vi "CLSUIP_ClearBlockDiagram.vi"(8 "error in (no error)":errorcluster, 11 "VI Refnum":refnum<vi>) -> (0 "error out":errorcluster, 3 "VI Refnum out":refnum<vi>)   [LabVIEW 2021, in "MemberVICreation.lvlib"]
uses:
  <resource>/Framework/Providers/LVClassLibrary/NewAccessors/MemberVICreation.lvlib
  <vilib>/Utility/miscctls.llb/LVPositionTypeDef.ctl
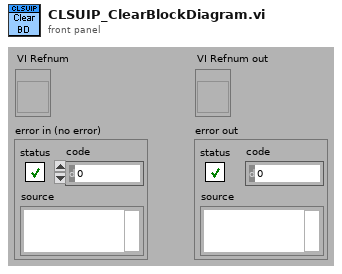
[diagram p1: front panel]
types:
  T1 = typedef "LVPositionTypeDef.ctl" = cluster{"Left":i32, "Top":i32}
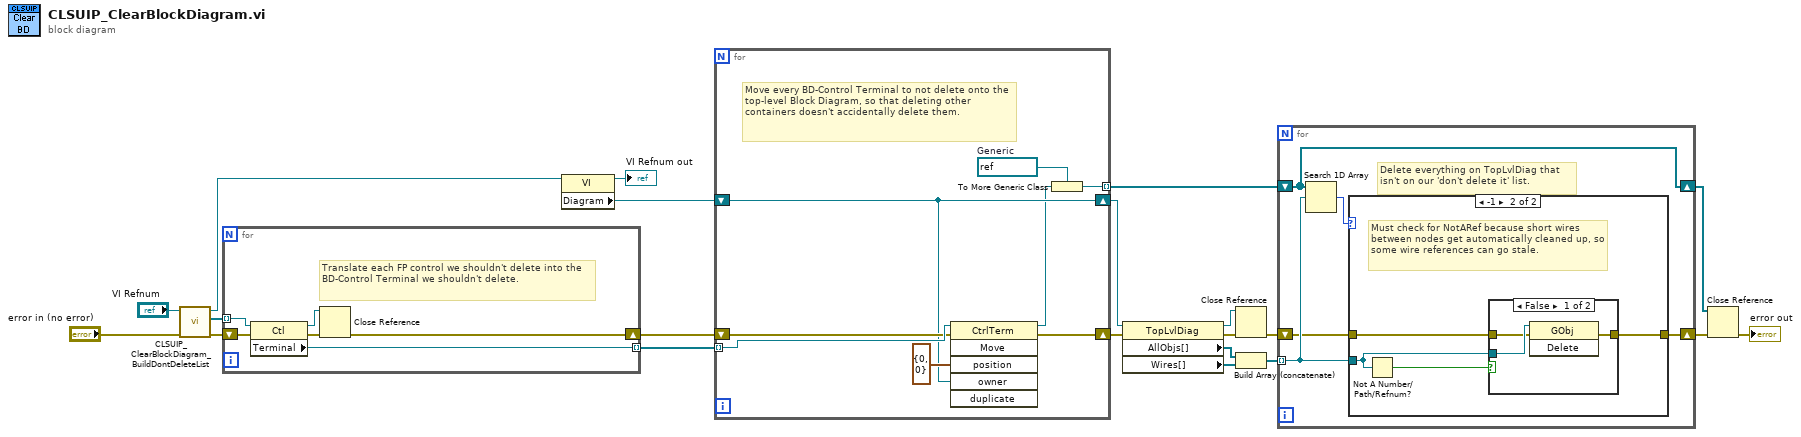
[diagram p0: block diagram]
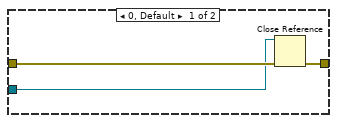
[diagram p2: hidden frame]
diagram:
  n1 = call <resource>:"CLSUIP_ClearBlockDiagram_BuildDontDeleteList.vi"("Error In"="error in (no error)", "VI Refnum In"="VI Refnum") -> ("Error Out"=w15:errorcluster, "Ctls which must not be deleted."=w16:refnum<vi>[], "VI Refnum Out"=w12:refnum<vi>)  [unwired: 7 in]
  n2 = for {
    tunnel: w16 -> [w27] mode=indexing
    tunnel: [w26] -> w13 mode=indexing
    shift-right: [w23] -> w14
    shift-left: w15 -> [w25]
    # "Translate each FP control we shouldn't delete into the BD-Control Terminal we shouldn't delete."
    n3 = property class="Ctl"(reference=w27, error in=w25) -> (reference out=w22:refnum<vi>, error out=w24:errorcluster, "Terminal"=w26:refnum<vi>)
    n4 = Close Reference(reference=w22, error in (no error)=w24) -> (error out=w23:errorcluster)
  }
  n5 = property class="VI"(reference=w12) -> (reference out=→"VI Refnum out":refnum<vi>, "Diagram"=w10:refnum<vi>)  [unwired: 1 in, 1 out]
  n6 = for {
    shift-right: [w32] -> w18
    shift-left: w14 -> [w33]
    tunnel: w13 -> [w34] mode=indexing
    tunnel: [w28] -> w5 mode=indexing
    shift-right: [w31] -> w9
    shift-left: w10 -> [w31]
    w29 = refnum<vi> refnum  # Generic
    # "Move every BD-Control Terminal to not delete onto the top-level Block Diagram, so that deleting other containers doesn't accidentally delete them."
    n7 = invoke class="CtrlTerm" method="Move"(reference=w34, error in=w33, "position"=T1 {"Left"=0, "Top"=0}, "owner"=w31) -> (reference out=w30:refnum<vi>, error out=w32:errorcluster)  [unwired: 2 in, 4 out]
    n8 = To More Generic Class(target class=w29, reference=w30) -> (generic class reference=w28:refnum<vi>)
  }
  n9 = property on="Property Node" class="TopLvlDiag"(reference=w9, error in=w18) -> (reference out=w20:refnum<vi>, error out=w17:errorcluster, "AllObjs[]"=w8:refnum<vi>[], "Wires[]"=w7:refnum<vi>[])
  n10 = Close Reference(reference=w20, error in (no error)=w17) -> (error out=w4:errorcluster)
  n11 = Build Array (concatenate)(w8, w7) -> (w6:refnum<vi>[])
  n12 = for {
    tunnel: w6 -> [w39] mode=indexing
    shift-right: [w36] -> w3
    shift-left: w5 -> [w36]
    shift-right: [w37] -> w2
    shift-left: w4 -> [w38]
    # "Delete everything on TopLvlDiag that isn't on our 'don't delete it' list."
    n13 = Search 1D Array(1D array=w36, element=w39) -> (index of element=w40:i32)  [unwired: 1 out]
    n14 = case shown="-1" w40 {
      tunnel: [w43 w47] -> w37
      tunnel: w39 -> [w41 w46]
      tunnel: w38 -> [w42 w44]
      frame 0, Default {
        n15 = Close Reference(reference=w41, error in (no error)=w42) -> (error out=w43:errorcluster)
      }
      frame -1 {
        # "Must check for NotARef because short wires between nodes get automatically cleaned up, so some wire references can go stale."
        n16 = Not A Number/Path/Refnum?(number/path/refnum=w46) -> (NaN/Path/Refnum?=w45:bool)
        n17 = case shown="False" w45 {
          tunnel: [w50 w51] -> w47
          tunnel: w46 -> [w49 _]
          tunnel: w44 -> [w48 w51]
          frame False {
            n18 = invoke on="Invoke Node" class="GObj" method="Delete"(reference=w49, error in=w48) -> (error out=w50:errorcluster)  [unwired: 1 in, 2 out]
          }
          frame True {
          }
        }
      }
    }
  }
  n19 = Close Reference(reference=w3, error in (no error)=w2) -> (error out=→"error out":errorcluster)
